vi "Sub Init Vi.vi"(8 "error in (no error)":errorcluster, 11 "IDE simple in":refnum<class "LF2R IDE.lvclass">) -> (0 "error out":errorcluster, 3 "IDE simple out":refnum<class "LF2R IDE.lvclass">)   [LabVIEW 2018, in "LF2R IDE.lvlib" / "LF2R IDE.lvclass"]
uses:
  LF2R IDE.lvclass
  LF2R IDE.lvclass/LF2R IDE.ctl
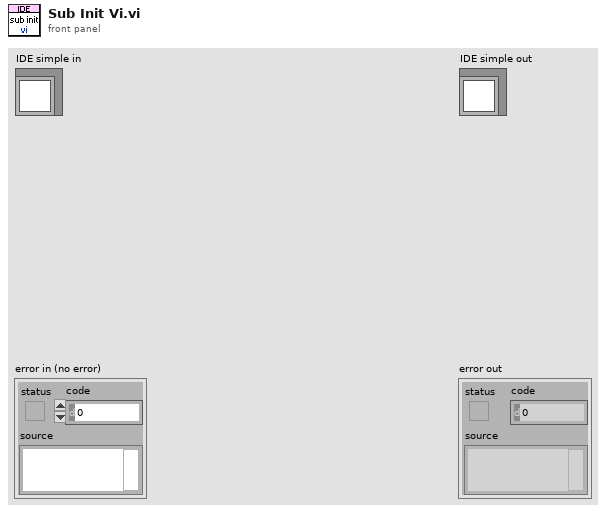
[diagram p1: front panel]
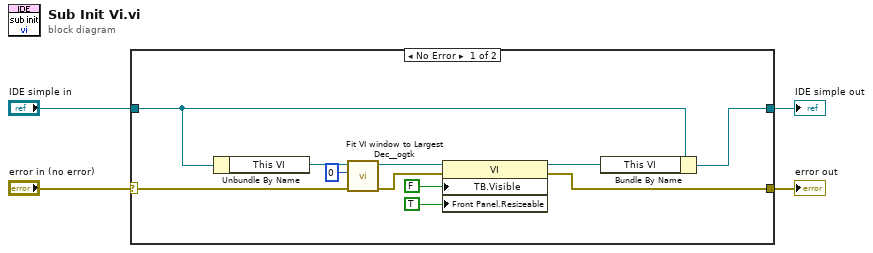
[diagram p0: block diagram]
diagram:
  n1 = case shown="No Error" "error in (no error)" {
    selector: "error in (no error)" -> [w8 w17]
    tunnel: [w7 w17] -> w3
    tunnel: [w6 w16] -> w1
    tunnel: "IDE simple in" -> [w10 w16]
    frame No Error {
      n2 = Unbundle By Name(w10) -> ("This VI"=w15:refnum<vi>)
      n3 = call <userlib>:"Fit VI window to Largest Dec__ogtk.vi"("error in (no error)"=w8, "border spacing (2 px)"=0, "VI Ref (calling VI)"=w15) -> ("error out"=w9:errorcluster, "dup VI Ref"=w13:refnum<vi>)  [unwired: 3 in]
      n4 = property class="VI"(reference=w13, error in=w9, "TB.Visible"=FALSE ("Tool Bar:Visible"), "Front Panel.Resizeable"=TRUE ("Front Panel Window:Resizable")) -> (reference out=w5:refnum<vi>, error out=w7:errorcluster)
      n5 = Bundle By Name(cluster=w10, "This VI"=w5) -> (w6:refnum<class "LF2R IDE.lvclass">)
    }
    frame Error {
    }
  }
  "error out" <- w3
  "IDE simple out" <- w1
